vi "GetImageBufferLength.vi"(8 "error in (no error)":errorcluster) -> (0 "error out":errorcluster, 2 "Image Buffer Length":i32)   [LabVIEW 2017, in "SystemController.lvclass"]
doc: "---------------------------------------------------------------\nJKI State Machine Objects™\nhttp://jki.net/state-machine-objects/\nCopyright (C) 2005-2015, JKI <info@jki.net>\nALL RIGHTS RESERVEDJKI State Machine Objects (SMO) 1.0.0.5\nJKI - JKI\nCopyright (c) 2016, JKI"
uses:
  SystemController.lvclass
panel:
  # "For instructions on how to use the JKI State Machine Objects, examples and video tutorials, visit:\nhttp://jki.net/state-machine-objects/\n\nJKI State Machine Objects™\nhttp://jki.net/state-machine-objects/\nCopyright (C) 2005-2015, JKI <info@jki.net>\nALL RIGHTS RESERVED"
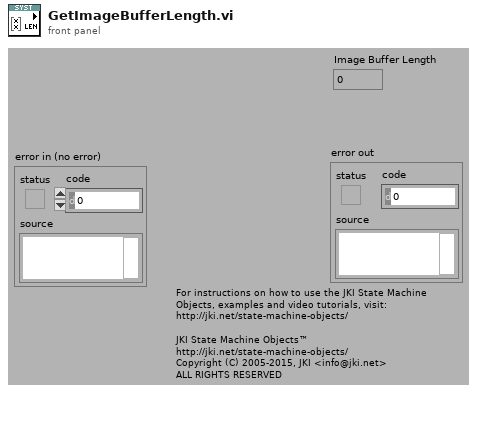
[diagram p1: front panel]
types:
  T1 = typedef "SystemController.lvclass/Configuration--Cluster.ctl" = cluster{"Camera":T2, "Find Eyes":bool, "Acquisition Rate (ms)":i32, "Image Buffer Length":i32}
  T2 = typedef "SystemController.lvclass/CameraConfig--Cluster.ctl" = cluster{"Simulate Camera":bool, "IMAQ Camera":T3, "Simulated Camera Image":path}
  T3 = typedef "Camera_IMAQdx.lvclass/Configuration--Cluster.ctl" = cluster{"Camera Interface Name":string, "Number of Buffers":u32, "Image Name":string, "Image Type":T4}
  T4 = typedef "Image Type" = u32
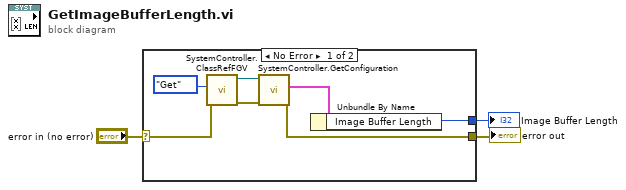
[diagram p0: block diagram]
diagram:
  n1 = case shown="No Error" "error in (no error)" {
    selector: "error in (no error)" -> [w6 w11]
    tunnel: [w7 w11] -> w3
    tunnel: [w4 _] -> w2
    frame No Error {
      n2 = call "SystemController.ClassRefFGV.vi"("error in (no error)"=w6, "Set/Get"=enum16{"Set", "Get"}."Get") -> ("error out"=w8:errorcluster, "SystemController out"=w9:refnum<class "SystemController.lvclass">)  [unwired: 8 in]
      n3 = call "SystemController.GetConfiguration.vi"("error in (no error)"=w8, "SystemController"=w9) -> ("error out"=w7:errorcluster, "Configuration"=w5:T1)  [unwired: 7 in, 1 out]
      n4 = Unbundle By Name(w5) -> ("Image Buffer Length"=w4:i32)
    }
    frame Error {
    }
  }
  "Image Buffer Length" <- w2
  "error out" <- w3
